vi "alpha_0.6.vi"() -> ()   [LabVIEW 2018]
panel:
  in  "day":dbl
  in  "func":string
  in  "path":path
  out "Congestionamento 2":bool
  in  "Rácio de entrada 2":dbl
  in  "Slide 2":dbl(slide) scale=0.0..10.0
  in  "Velocidade 2":dbl
  out "Vel3":bool
  out "Vel2":bool
  out "Vel1":bool
  out "RP1 3":bool
  out "GP1 3":bool
  out "G1 3":bool
  out "Y1 3":bool
  out "R1 3":bool
  out "RP1 2":bool
  out "GP1 2":bool
  out "G1 2":bool
  out "Y1 2":bool
  out "R1 2":bool
  out "RP1":bool
  out "GP1":bool
  out "G1":bool
  out "Y1":bool
  out "R1":bool
  in  "Rácio de entrada":dbl
  in  "Rácio de entrada 3":dbl
  out "Tempo no Vermelho":dbl caption="Elapsed Time (s)"
  out "Tempo no Verde + Amarelo":dbl caption="Elapsed Time (s)"
  out "Congestionamento 3":bool
  out "Congestionamento 1":bool
  in  "Slide 3":dbl(slide) scale=0.0..10.0
  in  "Slide 1":dbl(slide) scale=0.0..10.0
  in  "Caso de emergência":bool
  out "GreenP 2":bool
  out "RedP 2":bool
  out "GreenP 1":bool
  out "RedP 1":bool
  in  "Estado 2":dbl
  out "Velocidade excedida 3":bool
  in  "Velocidade 3":dbl
  out "RED 4":bool
  out "YELLOW 4":bool
  out "GREEN 4":bool
  out "Velocidade excedida 2":bool
  in  "Velocidade":dbl
  out "RED 3":bool
  out "YELLOW 3":bool
  out "GREEN 3":bool
  in  "stop":bool
  in  "Timer (s)":dbl
  # "Inputs"
  # "Inputs"
  # "Inputs"
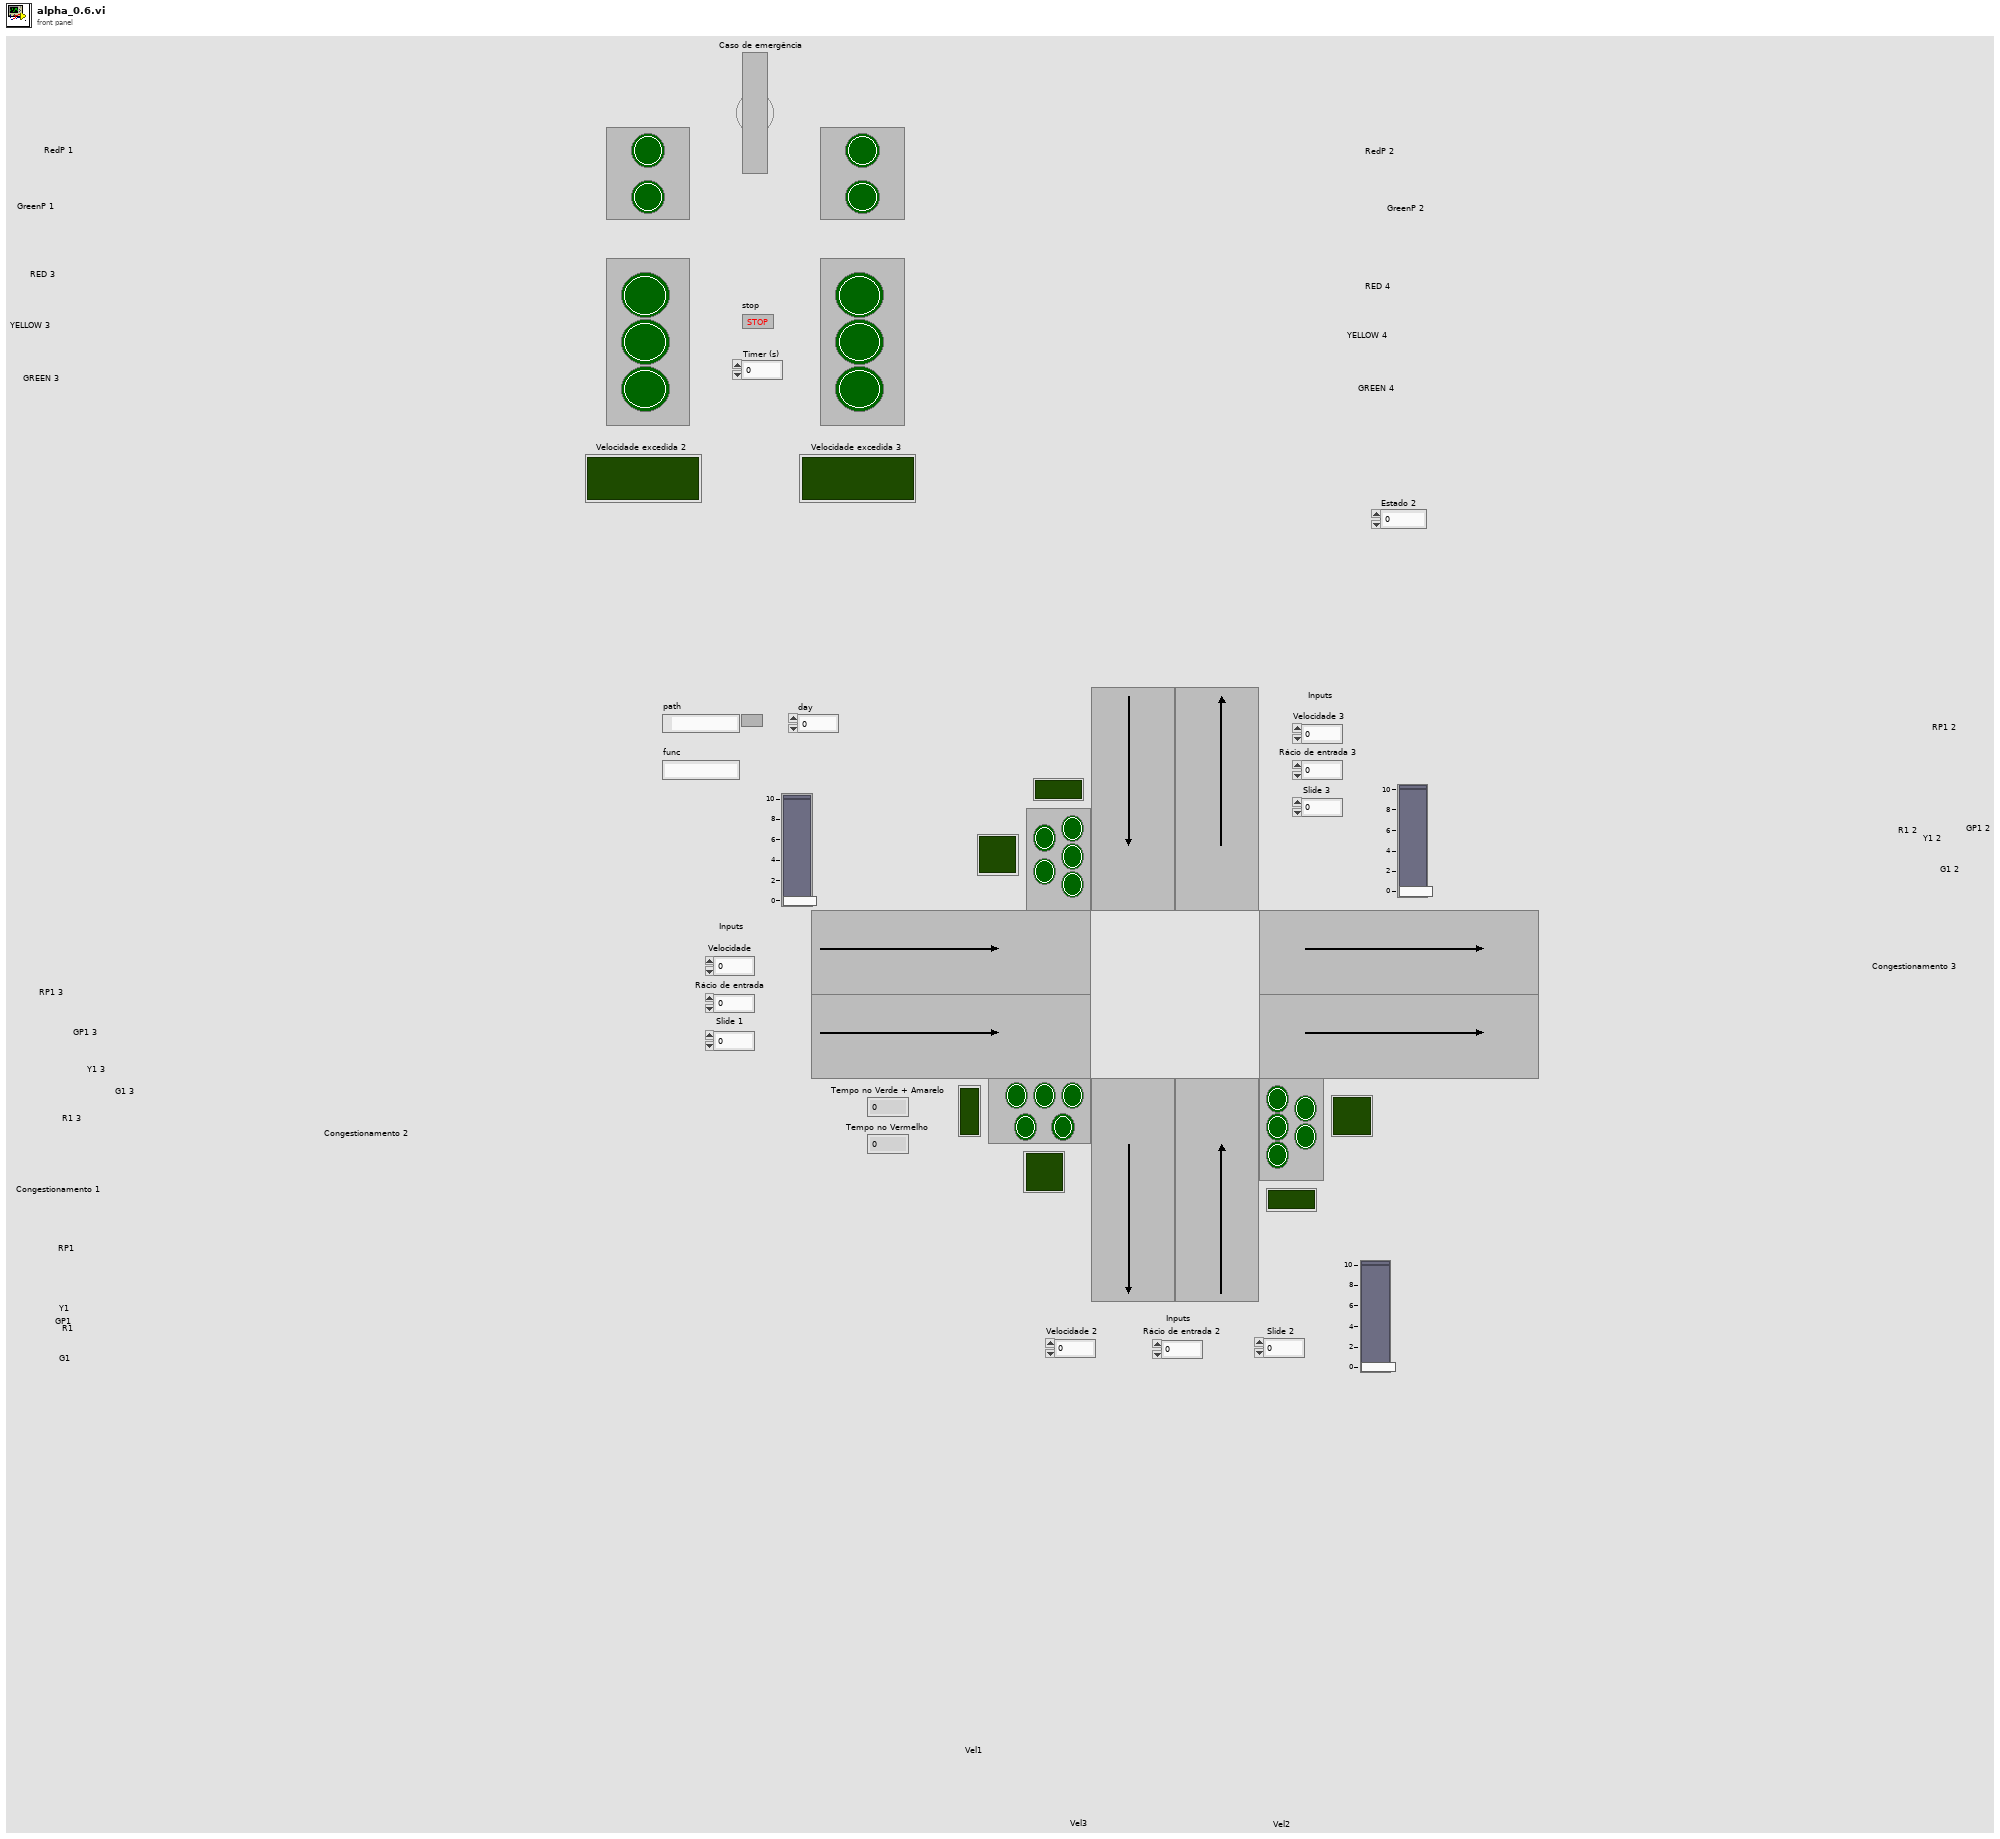
[diagram p1: front panel]
types:
  T1 = cluster{"return value[0]":dbl, "return value[1]":dbl, "return value[2]":dbl, "return value[3]":dbl, "return value[4]":dbl, "return value[5]":dbl, "return value[6]":dbl, "return value[7]":dbl, "return value[8]":dbl}
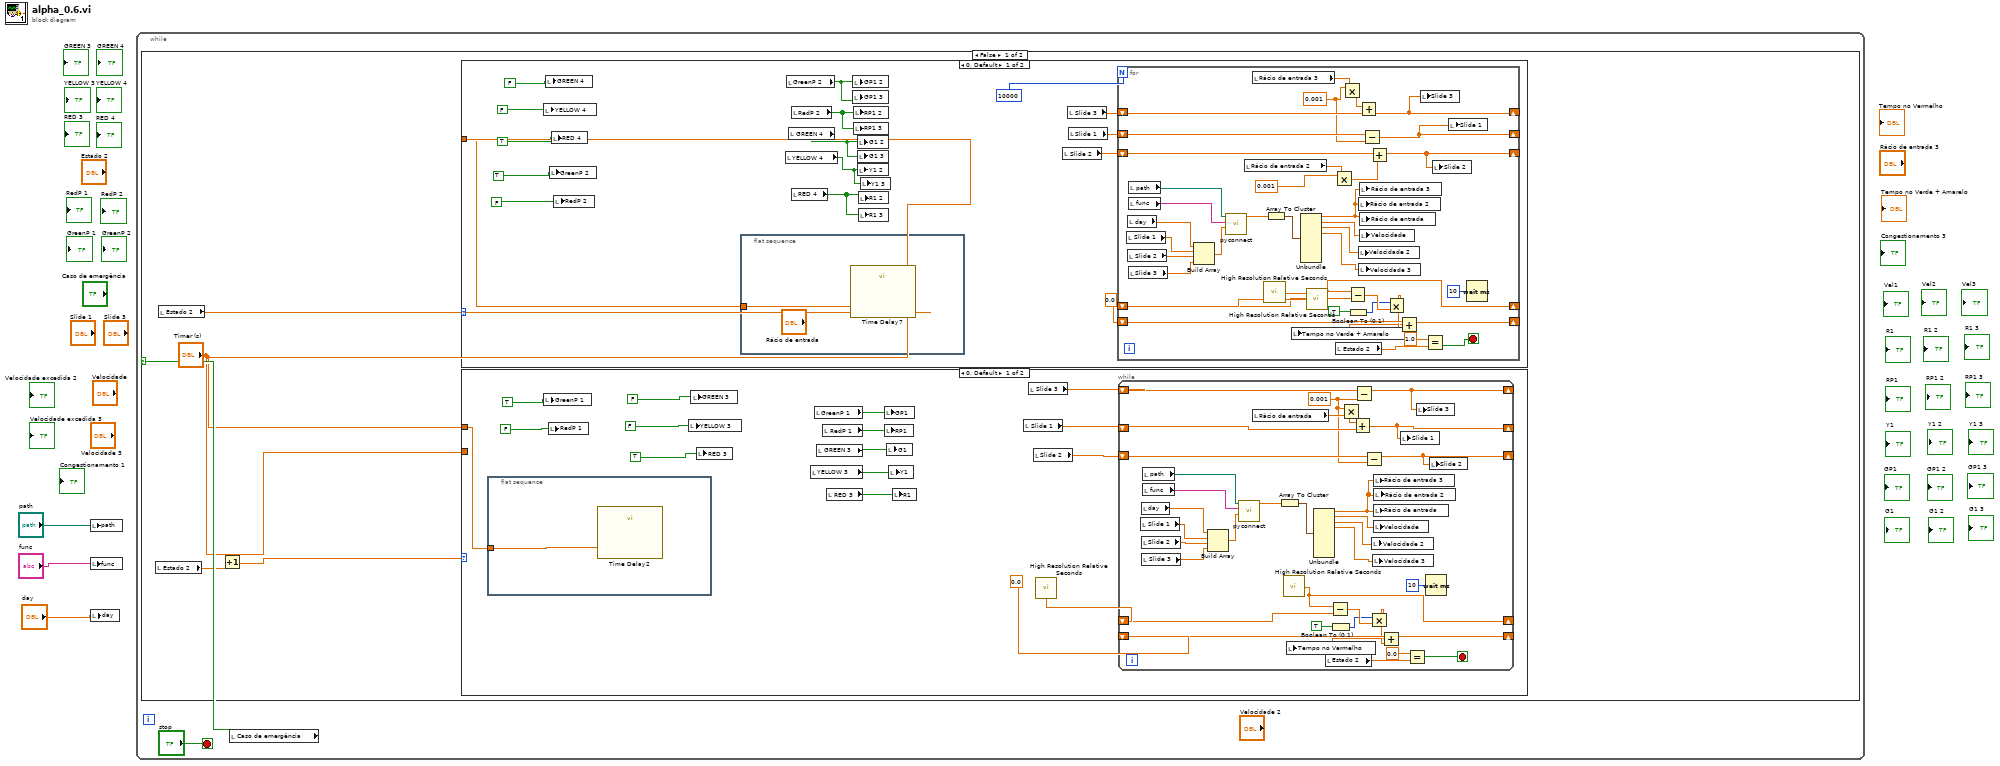
[diagram p0: block diagram]
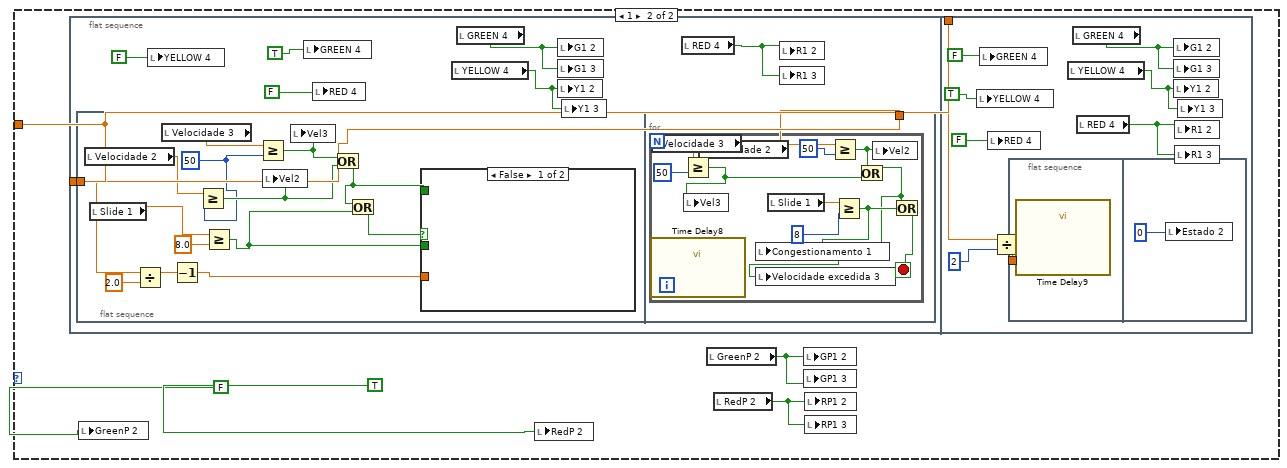
[diagram p2: hidden frame]
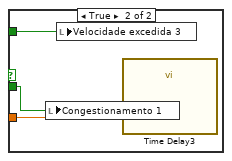
[diagram p3: hidden frame]
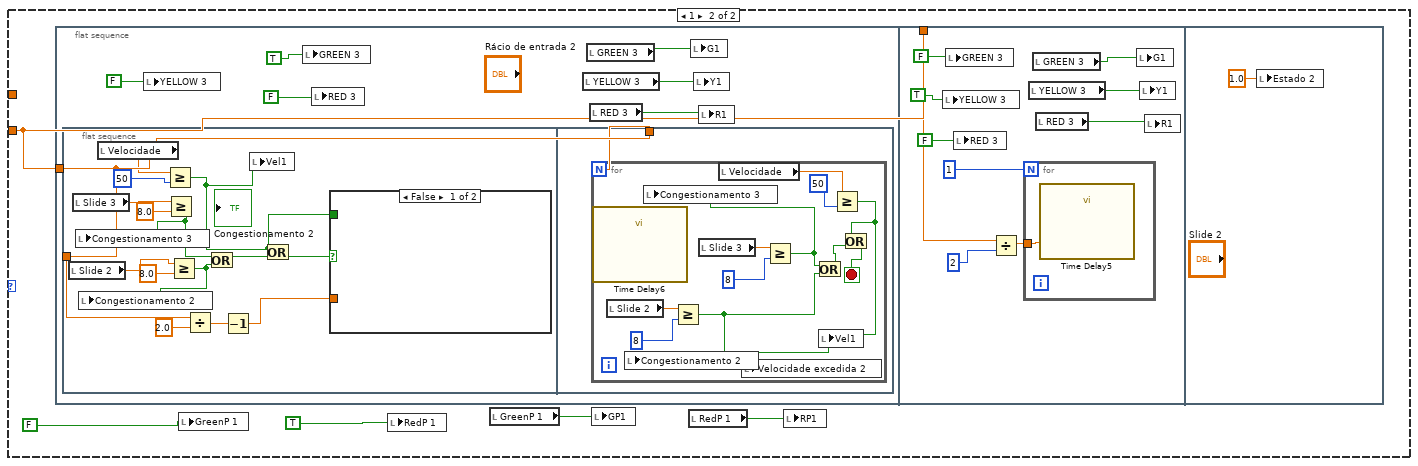
[diagram p4: hidden frame]
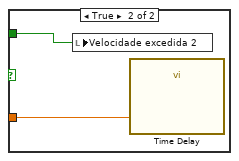
[diagram p5: hidden frame]
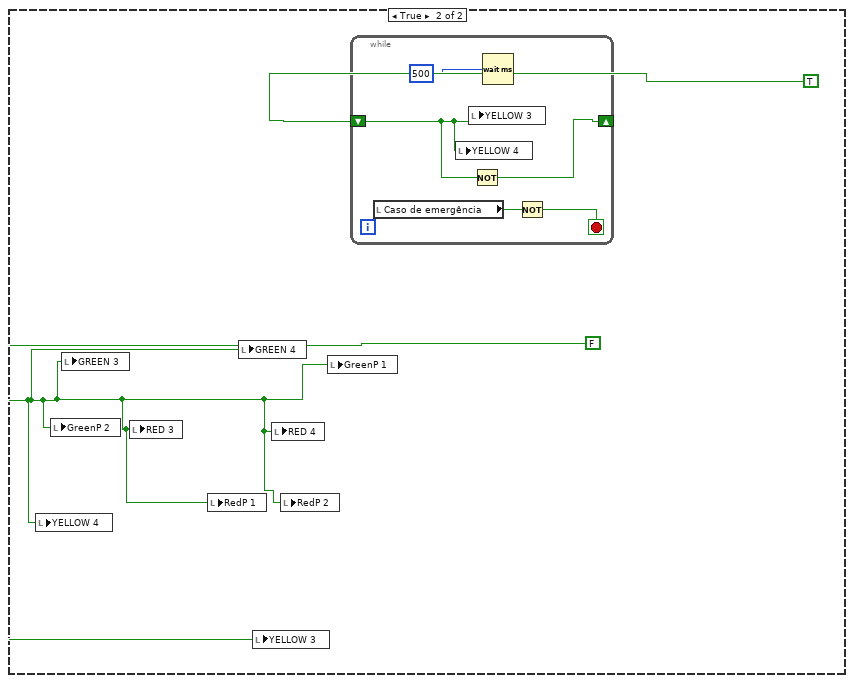
[diagram p6: hidden frame]
diagram:
  n1 = local write "path"("path") -> ()
  n2 = local write "func"("func") -> ()
  n3 = local write "day"("day") -> ()
  n4 = while {
    stop <- "stop" stop-if-true
    n5 = local read "Caso de emergência"() -> (w4:bool)
    n6 = case shown="False" w4 {
      frame False {
        n7 = local read "Estado 2"() -> (w9:dbl)
        n8 = local read "Estado 2"() -> (w7:dbl)
        n9 = Increment(x=w9) -> (x+1=w8:dbl)
        n10 = case shown="0, Default" w7 {
          tunnel: "Timer (s)" -> [w21 w69]
          frame 0, Default {
            n11 = local write "YELLOW 4"(FALSE) -> ()
            n12 = local write "GREEN 4"(FALSE) -> ()
            n13 = local write "GreenP 2"(TRUE) -> ()
            n14 = local write "RED 4"(TRUE) -> ()
            n15 = local write "RedP 2"(FALSE) -> ()
            n16 = flat-sequence {
              tunnel: w21 -> [w64]
              frame #0 {
                n17 = call "Time Delay7"("Delay Time (s)"=w64) -> ()  [unwired: 10 in, 1 out]
              }
            }
            n18 = local read "YELLOW 4"() -> (w12:bool)
            n19 = local read "GreenP 2"() -> (w15:bool)
            n20 = local read "GREEN 4"() -> (w13:bool)
            n21 = local read "RedP 2"() -> (w14:bool)
            n22 = local read "RED 4"() -> (w11:bool)
            n23 = local write "GP1 2"(w15) -> ()
            n24 = local write "GP1 3"(w15) -> ()
            n25 = local write "RP1 2"(w14) -> ()
            n26 = local write "RP1 3"(w14) -> ()
            n27 = local write "G1 2"(w13) -> ()
            n28 = local write "G1 3"(w13) -> ()
            n29 = local write "Y1 2"(w12) -> ()
            n30 = local write "R1 2"(w11) -> ()
            n31 = local write "R1 3"(w11) -> ()
            n32 = local write "Y1 3"(w12) -> ()
            n33 = local read "Slide 2"() -> (w10:dbl)
            n34 = local read "Slide 3"() -> (w16:dbl)
            n35 = local read "Slide 1"() -> (w17:dbl)
            n36 = call <vilib>:"High Resolution Relative Seconds.vi"() -> ("relative seconds"=w20:dbl)
            n37 = for {
              N: 10000 -> [_]
              shift-right: [w61] -> _
              shift-left: w20 -> [w62]
              shift-right: [w55] -> _
              shift-left: 0.0 -> [w60]
              shift-right: [w42] -> _
              shift-left: w16 -> [w51]
              shift-right: [w41] -> _
              shift-left: w17 -> [w48]
              shift-right: [w40] -> _
              shift-left: w10 -> [w46]
              stop <- w53 stop-if-true
              w47 = 0.001 ("x")
              n38 = local read "Slide 1"() -> (w35:dbl)
              n39 = local read "day"() -> (w36:dbl)
              n40 = local read "Slide 2"() -> (w34:dbl)
              n41 = local read "Slide 3"() -> (w33:dbl)
              n42 = local read "path"() -> (w39:path)
              n43 = local read "func"() -> (w38:string)
              n44 = Build Array(w36, w35, w34, w33) -> (w32:dbl[])
              n45 = call "pyconnect.vi"("Array"=w32, "function name"=w38, "module path"=w39) -> ("return value"=w31:dbl[])  [unwired: 8 in]
              n46 = local read "Rácio de entrada 2"() -> (w44:dbl)
              n47 = local read "Rácio de entrada 3"() -> (w50:dbl)
              n48 = call <vilib>:"High Resolution Relative Seconds.vi"() -> ("relative seconds"=w61:dbl)
              n49 = Array To Cluster(array=w31) -> (cluster=w37:T1)
              n50 = Unbundle(w37) -> ("return value[0]"=w27:dbl, "return value[1]"=w30:dbl, "return value[2]"=w29:dbl, "return value[3]"=w28:dbl)  [unwired: 5 out]
              n51 = Multiply(x=0.001, y=w44) -> (x*y=w43:dbl)
              n52 = local read "Estado 2"() -> (w54:dbl)
              n53 = Multiply(x=w47, y=w50) -> (x*y=w49:dbl)
              n54 = Subtract(x=w61, y=w62) -> (x-y=w58:dbl)
              n55 = Boolean To (0,1)(Boolean=TRUE) -> (0, 1=w56:i16)
              n56 = Add(x=w49, y=w51) -> (x+y=w42:dbl)
              n57 = local write "Velocidade 2"(w29) -> ()
              n58 = local write "Rácio de entrada 2"(w27) -> ()
              n59 = local write "Velocidade 3"(w28) -> ()
              n60 = local write "Rácio de entrada 3"(w27) -> ()
              n61 = local write "Rácio de entrada"(w27) -> ()
              n62 = local write "Velocidade"(w30) -> ()
              n63 = Subtract(x=w48, y=w47) -> (x-y=w41:dbl)
              n64 = Add(x=w46, y=w43) -> (x+y=w40:dbl)
              n65 = Multiply(x=w56, y=w58) -> (x*y=w57:dbl)
              n66 = Add(x=w60, y=w57) -> (x+y=w55:dbl)
              n67 = local write "Tempo no Verde + Amarelo"(w55) -> ()
              n68 = local write "Slide 3"(w42) -> ()
              n69 = Equal?(x=1.0, y=w54) -> (x = y?=w53:bool)
              n70 = local write "Slide 2"(w40) -> ()
              n71 = local write "Slide 1"(w41) -> ()
              n72 = Wait (ms)(milliseconds to wait=u32 10) -> ()  [unwired: 1 out]
            }
          }
          frame 1 {
            n73 = flat-sequence {
              tunnel: w69 -> [w73]
              tunnel: w69 -> [w110]
              frame #0 {
                n74 = flat-sequence {
                  tunnel: w73 -> [w86]
                  tunnel: w73 -> [w94]
                  frame #0 {
                    w77 = 50
                    n75 = local read "Velocidade 2"() -> (w79:dbl)
                    n76 = local read "Slide 1"() -> (w83:dbl)
                    n77 = Divide(x=w86, y=2.0) -> (x/y=w89:dbl)
                    n78 = local read "Velocidade 3"() -> (w88:dbl)
                    n79 = Decrement(x=w89) -> (x-1=w90:dbl)
                    n80 = Greater Or Equal?(x=w79, y=w77) -> (x >= y?=w78:bool)
                    n81 = Greater Or Equal?(x=w83, y=8.0) -> (x >= y?=w81:bool)
                    n82 = Greater Or Equal?(x=w88, y=w77) -> (x >= y?=w82:bool)
                    n83 = local write "Vel2"(w78) -> ()
                    n84 = local write "Vel3"(w82) -> ()
                    n85 = Or(x=w82, y=w78) -> (x .or. y?=w80:bool)
                    n86 = Or(x=w80, y=w81) -> (x .or. y?=w84:bool)
                    n87 = case shown="False" w84 {
                      tunnel: w90 -> [_ w93]
                      tunnel: w80 -> [_ w91]
                      tunnel: w81 -> [_ w92]
                      frame False {
                      }
                      frame True {
                        n88 = local write "Congestionamento 1"(w92) -> ()
                        n89 = local write "Velocidade excedida 3"(w91) -> ()
                        n90 = call "Time Delay3"("Delay Time (s)"=w93) -> ()  [unwired: 10 in, 1 out]
                      }
                    }
                  }
                  frame #1 {
                    n91 = for {
                      N: w94 -> [_]
                      stop <- w103 stop-if-true
                      n92 = call "Time Delay8"() -> ()  [unwired: 11 in, 1 out]
                      n93 = local read "Velocidade 3"() -> (w105:dbl)
                      n94 = Greater Or Equal?(x=w105, y=50) -> (x >= y?=w99:bool)
                      n95 = local write "Vel3"(w99) -> ()
                      n96 = local read "Velocidade 2"() -> (w97:dbl)
                      n97 = local read "Slide 1"() -> (w102:dbl)
                      n98 = Greater Or Equal?(x=w97, y=50) -> (x >= y?=w95:bool)
                      n99 = Greater Or Equal?(x=w102, y=8) -> (x >= y?=w100:bool)
                      n100 = local write "Congestionamento 1"(w100) -> ()
                      n101 = Or(x=w95, y=w99) -> (x .or. y?=w98:bool)
                      n102 = local write "Velocidade excedida 3"(w98) -> ()
                      n103 = local write "Vel2"(w95) -> ()
                      n104 = Or(x=w98, y=w100) -> (x .or. y?=w103:bool)
                    }
                  }
                }
                n105 = local write "YELLOW 4"(FALSE) -> ()
                n106 = local write "GREEN 4"(TRUE) -> ()
                n107 = local write "RED 4"(FALSE) -> ()
                n108 = local read "YELLOW 4"() -> (w71:bool)
                n109 = local read "GREEN 4"() -> (w72:bool)
                n110 = local write "G1 2"(w72) -> ()
                n111 = local write "G1 3"(w72) -> ()
                n112 = local write "Y1 2"(w71) -> ()
                n113 = local write "Y1 3"(w71) -> ()
                n114 = local read "RED 4"() -> (w70:bool)
                n115 = local write "R1 2"(w70) -> ()
                n116 = local write "R1 3"(w70) -> ()
              }
              frame #1 {
                n117 = local write "YELLOW 4"(TRUE) -> ()
                n118 = local write "GREEN 4"(FALSE) -> ()
                n119 = local write "RED 4"(FALSE) -> ()
                n120 = Divide(x=w110, y=2) -> (x/y=w109:dbl)
                n121 = flat-sequence {
                  tunnel: w109 -> [w115]
                  frame #0 {
                    n122 = call "Time Delay9"("Delay Time (s)"=w115) -> ()  [unwired: 10 in, 1 out]
                  }
                  frame #1 {
                    n123 = local write "Estado 2"(0) -> ()
                  }
                }
                n124 = local read "YELLOW 4"() -> (w107:bool)
                n125 = local read "GREEN 4"() -> (w108:bool)
                n126 = local read "RED 4"() -> (w106:bool)
                n127 = local write "G1 2"(w108) -> ()
                n128 = local write "G1 3"(w108) -> ()
                n129 = local write "Y1 2"(w107) -> ()
                n130 = local write "R1 2"(w106) -> ()
                n131 = local write "R1 3"(w106) -> ()
                n132 = local write "Y1 3"(w107) -> ()
              }
            }
            n133 = local write "GreenP 2"(FALSE) -> ()
            n134 = local write "RedP 2"(TRUE) -> ()
            n135 = local read "GreenP 2"() -> (w66:bool)
            n136 = local read "RedP 2"() -> (w65:bool)
            n137 = local write "GP1 2"(w66) -> ()
            n138 = local write "GP1 3"(w66) -> ()
            n139 = local write "RP1 2"(w65) -> ()
            n140 = local write "RP1 3"(w65) -> ()
          }
        }
        n141 = case shown="0, Default" w8 {
          tunnel: "Timer (s)" -> [_ w170]
          tunnel: "Timer (s)" -> [w124 _]
          frame 0, Default {
            n142 = flat-sequence {
              tunnel: w124 -> [w133]
              frame #0 {
                n143 = call "Time Delay2"("Delay Time (s)"=w133) -> ()  [unwired: 10 in, 1 out]
              }
            }
            n144 = local write "GreenP 1"(TRUE) -> ()
            n145 = local write "RedP 1"(FALSE) -> ()
            n146 = local write "YELLOW 3"(FALSE) -> ()
            n147 = local write "GREEN 3"(FALSE) -> ()
            n148 = local write "RED 3"(TRUE) -> ()
            n149 = local read "YELLOW 3"() -> (w119:bool)
            n150 = local read "GreenP 1"() -> (w122:bool)
            n151 = local read "GREEN 3"() -> (w120:bool)
            n152 = local read "RedP 1"() -> (w121:bool)
            n153 = local read "RED 3"() -> (w118:bool)
            n154 = local write "GP1"(w122) -> ()
            n155 = local write "RP1"(w121) -> ()
            n156 = local write "G1"(w120) -> ()
            n157 = local write "Y1"(w119) -> ()
            n158 = local write "R1"(w118) -> ()
            n159 = local read "Slide 1"() -> (w123:dbl)
            n160 = local read "Slide 3"() -> (w125:dbl)
            n161 = local read "Slide 2"() -> (w117:dbl)
            n162 = call <vilib>:"High Resolution Relative Seconds.vi"() -> ("relative seconds"=w127:dbl)
            n163 = while {
              shift-right: [w165] -> _
              shift-left: w127 -> [w166]
              shift-right: [w159] -> _
              shift-left: 0.0 -> [w164]
              shift-right: [w147] -> _
              shift-left: w125 -> [w155]
              shift-right: [w148] -> _
              shift-left: w123 -> [w152]
              shift-right: [w149] -> _
              shift-left: w117 -> [w151]
              stop <- w157 stop-if-true
              w150 = 0.001 ("y")
              n164 = local read "Slide 1"() -> (w139:dbl)
              n165 = local read "day"() -> (w138:dbl)
              n166 = local read "Slide 2"() -> (w140:dbl)
              n167 = local read "Slide 3"() -> (w141:dbl)
              n168 = local read "path"() -> (w135:path)
              n169 = local read "func"() -> (w136:string)
              n170 = Build Array(w138, w139, w140, w141) -> (w142:dbl[])
              n171 = call "pyconnect.vi"("Array"=w142, "function name"=w136, "module path"=w135) -> ("return value"=w143:dbl[])  [unwired: 8 in]
              n172 = local read "Rácio de entrada"() -> (w154:dbl)
              n173 = Array To Cluster(array=w143) -> (cluster=w137:T1)
              n174 = call <vilib>:"High Resolution Relative Seconds.vi"() -> ("relative seconds"=w165:dbl)
              n175 = Unbundle(w137) -> ("return value[0]"=w134:dbl, "return value[1]"=w144:dbl, "return value[2]"=w145:dbl, "return value[3]"=w146:dbl)  [unwired: 5 out]
              n176 = local read "Estado 2"() -> (w158:dbl)
              n177 = Subtract(x=w165, y=w166) -> (x-y=w162:dbl)
              n178 = Boolean To (0,1)(Boolean=TRUE) -> (0, 1=w160:i16)
              n179 = Multiply(x=w150, y=w154) -> (x*y=w153:dbl)
              n180 = Add(x=w153, y=w152) -> (x+y=w148:dbl)
              n181 = Subtract(x=w155, y=w150) -> (x-y=w147:dbl)
              n182 = Subtract(x=w151, y=w150) -> (x-y=w149:dbl)
              n183 = Multiply(x=w160, y=w162) -> (x*y=w161:dbl)
              n184 = local write "Velocidade 2"(w145) -> ()
              n185 = local write "Velocidade 3"(w146) -> ()
              n186 = local write "Rácio de entrada 3"(w134) -> ()
              n187 = local write "Rácio de entrada"(w134) -> ()
              n188 = local write "Velocidade"(w144) -> ()
              n189 = local write "Rácio de entrada 2"(w134) -> ()
              n190 = Add(x=w164, y=w161) -> (x+y=w159:dbl)
              n191 = local write "Tempo no Vermelho"(w159) -> ()
              n192 = local write "Slide 1"(w148) -> ()
              n193 = Equal?(x=0.0, y=w158) -> (x = y?=w157:bool)
              n194 = local write "Slide 3"(w147) -> ()
              n195 = Wait (ms)(milliseconds to wait=u32 10) -> ()  [unwired: 1 out]
              n196 = local write "Slide 2"(w149) -> ()
            }
          }
          frame 1 {
            n197 = flat-sequence {
              tunnel: w170 -> [w176]
              tunnel: w170 -> [w212]
              frame #0 {
                n198 = flat-sequence {
                  tunnel: w176 -> [w192]
                  tunnel: w176 -> [w197]
                  frame #0 {
                    n199 = local read "Slide 2"() -> (w180:dbl)
                    n200 = local read "Slide 3"() -> (w187:dbl)
                    n201 = local read "Velocidade"() -> (w194:dbl)
                    n202 = Greater Or Equal?(x=w194, y=50) -> (x >= y?=w185:bool)
                    n203 = Greater Or Equal?(x=w187, y=8.0) -> (x >= y?=w184:bool)
                    n204 = local write "Congestionamento 3"(w184) -> ()
                    n205 = Greater Or Equal?(x=w180, y=8.0) -> (x >= y?=w181:bool)
                    n206 = local write "Congestionamento 2"(w181) -> ()
                    n207 = Divide(x=w192, y=2.0) -> (x/y=w191:dbl)
                    n208 = Or(x=w184, y=w181) -> (x .or. y?=w183:bool)
                    n209 = Decrement(x=w191) -> (x-1=w189:dbl)
                    n210 = local write "Vel1"(w185) -> ()
                    n211 = Or(x=w185, y=w183) -> (x .or. y?=w188:bool)
                    n212 = case shown="False" w188 {
                      tunnel: w189 -> [_ w196]
                      tunnel: w185 -> [_ w195]
                      frame False {
                      }
                      frame True {
                        n213 = local write "Velocidade excedida 2"(w195) -> ()
                        n214 = call "Time Delay"("Delay Time (s)"=w196) -> ()  [unwired: 10 in, 1 out]
                      }
                    }
                  }
                  frame #1 {
                    n215 = for {
                      N: w197 -> [_]
                      stop <- w204 stop-if-true
                      n216 = call "Time Delay6"() -> ()  [unwired: 11 in, 1 out]
                      n217 = local read "Slide 2"() -> (w201:dbl)
                      n218 = Greater Or Equal?(x=w201, y=8) -> (x >= y?=w198:bool)
                      n219 = local write "Congestionamento 2"(w198) -> ()
                      n220 = local read "Slide 3"() -> (w206:dbl)
                      n221 = local read "Velocidade"() -> (w208:dbl)
                      n222 = Greater Or Equal?(x=w206, y=8) -> (x >= y?=w199:bool)
                      n223 = local write "Congestionamento 3"(w199) -> ()
                      n224 = Or(x=w199, y=w198) -> (x .or. y?=w200:bool)
                      n225 = Greater Or Equal?(x=w208, y=50) -> (x >= y?=w203:bool)
                      n226 = local write "Velocidade excedida 2"(w203) -> ()
                      n227 = local write "Vel1"(w203) -> ()
                      n228 = Or(x=w203, y=w200) -> (x .or. y?=w204:bool)
                    }
                  }
                }
                n229 = local write "YELLOW 3"(FALSE) -> ()
                n230 = local write "GREEN 3"(TRUE) -> ()
                n231 = local write "RED 3"(FALSE) -> ()
                n232 = local read "YELLOW 3"() -> (w174:bool)
                n233 = local read "GREEN 3"() -> (w175:bool)
                n234 = local read "RED 3"() -> (w173:bool)
                n235 = local write "G1"(w175) -> ()
                n236 = local write "Y1"(w174) -> ()
                n237 = local write "R1"(w173) -> ()
              }
              frame #1 {
                n238 = local write "YELLOW 3"(TRUE) -> ()
                n239 = local write "GREEN 3"(FALSE) -> ()
                n240 = local write "RED 3"(FALSE) -> ()
                n241 = Divide(x=w212, y=2) -> (x/y=w215:dbl)
                n242 = for {
                  N: 1 -> [_]
                  tunnel: w215 -> [w219]
                  n243 = call "Time Delay5"("Delay Time (s)"=w219) -> ()  [unwired: 10 in, 1 out]
                }
                n244 = local read "YELLOW 3"() -> (w211:bool)
                n245 = local read "GREEN 3"() -> (w209:bool)
                n246 = local read "RED 3"() -> (w210:bool)
                n247 = local write "G1"(w209) -> ()
                n248 = local write "Y1"(w211) -> ()
                n249 = local write "R1"(w210) -> ()
              }
              frame #2 {
                n250 = local write "Estado 2"(1.0 ("Estado 2")) -> ()
              }
            }
            n251 = local write "GreenP 1"(FALSE) -> ()
            n252 = local write "RedP 1"(TRUE) -> ()
            n253 = local read "GreenP 1"() -> (w168:bool)
            n254 = local write "GP1"(w168) -> ()
            n255 = local read "RedP 1"() -> (w169:bool)
            n256 = local write "RP1"(w169) -> ()
          }
        }
      }
      frame True {
        w221 = FALSE
        n257 = local write "YELLOW 4"(w221) -> ()
        n258 = local write "GreenP 2"(w221) -> ()
        n259 = local write "GREEN 3"(w221) -> ()
        n260 = local write "RED 3"(w221) -> ()
        n261 = local write "RedP 1"(w221) -> ()
        n262 = local write "GREEN 4"(w221) -> ()
        n263 = local write "YELLOW 3"(w221) -> ()
        n264 = local write "RED 4"(w221) -> ()
        n265 = local write "RedP 2"(w221) -> ()
        n266 = local write "GreenP 1"(w221) -> ()
        n267 = while {
          shift-right: [w227] -> _
          shift-left: TRUE -> [w223]
          stop <- w224 stop-if-true
          n268 = local read "Caso de emergência"() -> (w225:bool)
          n269 = local write "YELLOW 4"(w223) -> ()
          n270 = local write "YELLOW 3"(w223) -> ()
          n271 = Not(x=w223) -> (.not. x?=w227:bool)
          n272 = Wait (ms)(milliseconds to wait=500) -> ()  [unwired: 1 out]
          n273 = Not(x=w225) -> (.not. x?=w224:bool)
        }
      }
    }
  }
